vi "Add Label with Parameters.vi"(8 "error in":errorcluster, 10 "label":T2, 11 "port ref":T1 format="%.0x") -> (0 "error out":errorcluster, 3 "port ref out":T1 format="%.0x")   [LabVIEW 2020, in "Ballard ARINC 429 Scripting.lvlib"]
doc: "For Rx labels, this VI assumes SDI, SSM, and Parity have already been added as parameters if desired. For Tx labels, this VI automatically adds trigger channel for acyclic labels or disable channel for scheduled labels."
uses:
  Ballard ARINC 429 Scripting.lvlib
  <vilib>/NI VeriStand/Custom Device API/Custom Device Item Ref.ctl
  Shared/VS Channels Definition for Label.ctl
  Shared/VS Channel Definition for Parameter.ctl
  Shared/Parameter Definition.ctl
  <vilib>/NI/NI VeriStand Encoding and Decoding/Encoding.ctl
  Shared/Transfer Type.ctl
  Shared/SDI.ctl
  <vilib>/NI VeriStand/Custom Device API/Custom Device API.lvlib
  <vilib>/NI/NI VeriStand Encoding and Decoding/Encoding and Decoding.lvlib
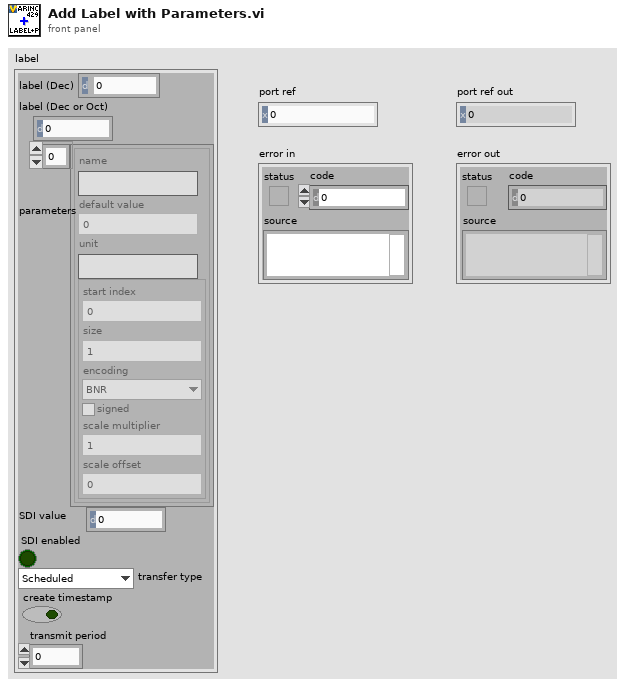
[diagram p1: front panel]
types:
  T1 = typedef "Custom Device API.lvlib/Custom Device Item Ref.ctl" = u64
  T2 = typedef "VS Channels Definition for Label.ctl" = cluster{"label (Dec)":u32, "label (Dec or Oct)":u32, "parameters":T3[], "SDI value":u8, "SDI enabled":bool, "transfer type":T6, "create timestamp":bool, "transmit period":u32}
  T3 = typedef "VS Channel Definition for Parameter.ctl" = cluster{"name":string, "default value":dbl, "unit":string, "Parameter":T4}
  T4 = typedef "Parameter Definition.ctl" = cluster{"start index":i32, "size":i32, "encoding":T5, "signed":bool, "scale multiplier":dbl, "scale offset":dbl}
  T5 = typedef "Encoding and Decoding.lvlib/Encoding.ctl" = enum16{"BNR", "BCD", "Discrete"}
  T6 = typedef "Transfer Type.ctl" = enum16{"Scheduled", "Acyclic", "Block", "Strobe"}
  T7 = cluster{"name":string, "unit":string, "default value":dbl}
  T8 = typedef "Direction.ctl" = enum16{"Rx", "Tx"}
  T9 = cluster{"SDI":bool, "SSM":bool, "Parity":bool, "Timestamp":bool}
  T10 = typedef "SDI.ctl" = i32
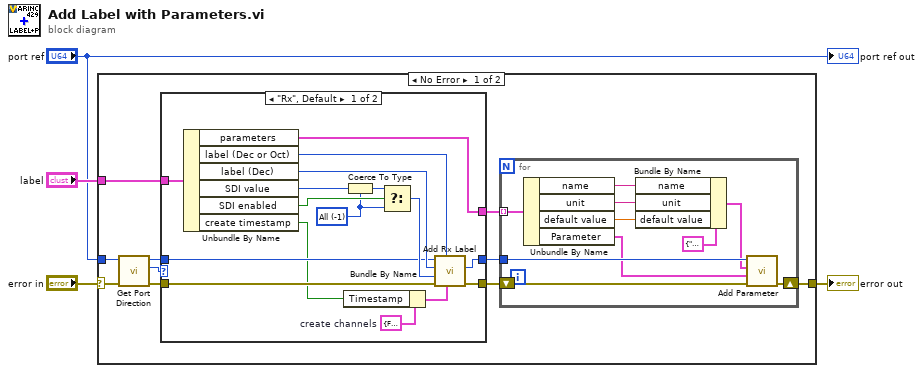
[diagram p0: block diagram]
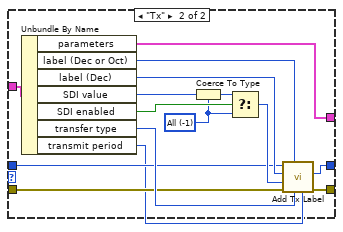
[diagram p2: hidden frame]
diagram:
  n1 = case shown="No Error" "error in" {
    selector: "error in" -> [w9 w56]
    tunnel: "port ref" -> [w7 _]
    tunnel: [w14 w56] -> w4
    tunnel: "label" -> [w13 _]
    frame No Error {
      n2 = call "Get Port Direction.vi"("error in"=w9, "port ref in"=w7) -> ("error out"=w6:errorcluster, "direction"=w5:T8, "port ref out"=w8:T1)  [unwired: 7 in]
      n3 = case shown="\"Rx\", Default" w5 {
        tunnel: w13 -> [w30 w45]
        tunnel: [w16 w32] -> w12
        tunnel: [w20 w37] -> w11
        tunnel: [w21 w36] -> w10
        tunnel: w8 -> [w23 w35]
        tunnel: w6 -> [w22 w34]
        frame "Rx", Default {
          w19 = T9 {"SDI"=FALSE, "SSM"=FALSE, "Parity"=FALSE, "Timestamp"=FALSE}  # create channels
          w26 = T10 -1 items=["All"=-1, "0 (b00)"=0, "1 (b01)"=1, "2 (b10)"=2, "3 (b11)"=3] ("SDI value")
          n4 = Unbundle By Name(w30) -> ("parameters"=w16:T3[], "label (Dec or Oct)"=w15:u32, "label (Dec)"=w24:u32, "SDI value"=w28:u8, "SDI enabled"=w29:bool, "create timestamp"=w18:bool)
          n5 = Bundle By Name(cluster=w19, "Timestamp"=w18) -> (w17:T9)
          n6 = Coerce To Type(0:w28, 1:w26) -> (2:w27:T10)
          n7 = Select(t=w27, s=w29, f=w26) -> (s? t:f=w25:T10)
          n8 = call "Add Rx Label.vi"("create channels"=w17, "label (Dec or Oct)"=w15, "error in"=w22, "SDI value"=w25, "label (Dec)"=w24, "port in"=w23) -> ("error out"=w20:errorcluster, "label"=w21:T1)  [unwired: 3 in, 1 out]
        }
        frame "Tx" {
          w41 = T10 -1 items=["All"=-1, "0 (b00)"=0, "1 (b01)"=1, "2 (b10)"=2, "3 (b11)"=3] ("SDI value")
          n9 = Unbundle By Name(w45) -> ("parameters"=w32:T3[], "label (Dec or Oct)"=w31:u32, "label (Dec)"=w38:u32, "SDI value"=w43:u8, "SDI enabled"=w44:bool, "transfer type"=w39:T6, "transmit period"=w33:u32)
          n10 = Coerce To Type(0:w43, 1:w41) -> (2:w42:T10)
          n11 = Select(t=w42, s=w44, f=w41) -> (s? t:f=w40:T10)
          n12 = call "Add Tx Label.vi"("scheduled transmit period (us)"=w33, "transfer type"=w39, "label (Dec or Oct)"=w31, "error in"=w34, "SDI value"=w40, "label (Dec)"=w38, "port in"=w35) -> ("error out"=w37:errorcluster, "label"=w36:T1)  [unwired: 2 in, 1 out]
        }
      }
      n13 = for {
        shift-right: [w53] -> w14
        shift-left: w11 -> [w54]
        tunnel: w12 -> [w52] mode=indexing
        tunnel: w10 -> [w55]
        n14 = Unbundle By Name(w52) -> ("name"=w49:string, "unit"=w48:string, "default value"=w47:dbl, "Parameter"=w51:T4)
        n15 = Bundle By Name(cluster=T7 {"name"="", "unit"="", "default value"=0.0} ("parameter"), "name"=w49, "unit"=w48, "default value"=w47) -> (w46:T7)
        n16 = call "Add Parameter.vi"("error in"=w54, "parameter encoding"=w51, "parameter definition"=w46, "label in"=w55) -> ("error out"=w53:errorcluster)  [unwired: 5 in, 2 out]
      }
    }
    frame Error {
    }
  }
  "error out" <- w4
  "port ref out" <- "port ref"
